vi "edge_trig_setup.vi"(7 "Tigger Level":dbl, 8 "error in (no error)":errorcluster, 9 "Coupling":u32(slide) scale=0.0..1.0, 10 "Channel":u32(slide)=1 scale=1.0..2.0, 11 "VISA In":refnum<visa-resource-name>) -> (0 "error out":errorcluster, 3 "VISA Out":refnum<visa-resource-name>)   [LabVIEW 2011]
panel:
  out "String Sent":string
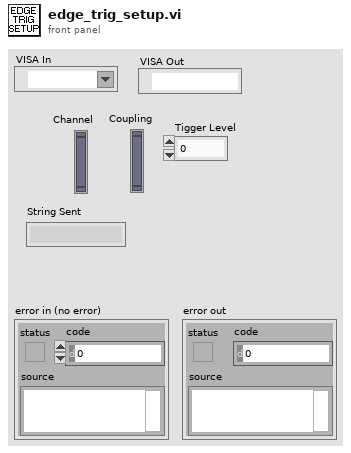
[diagram p1: front panel]
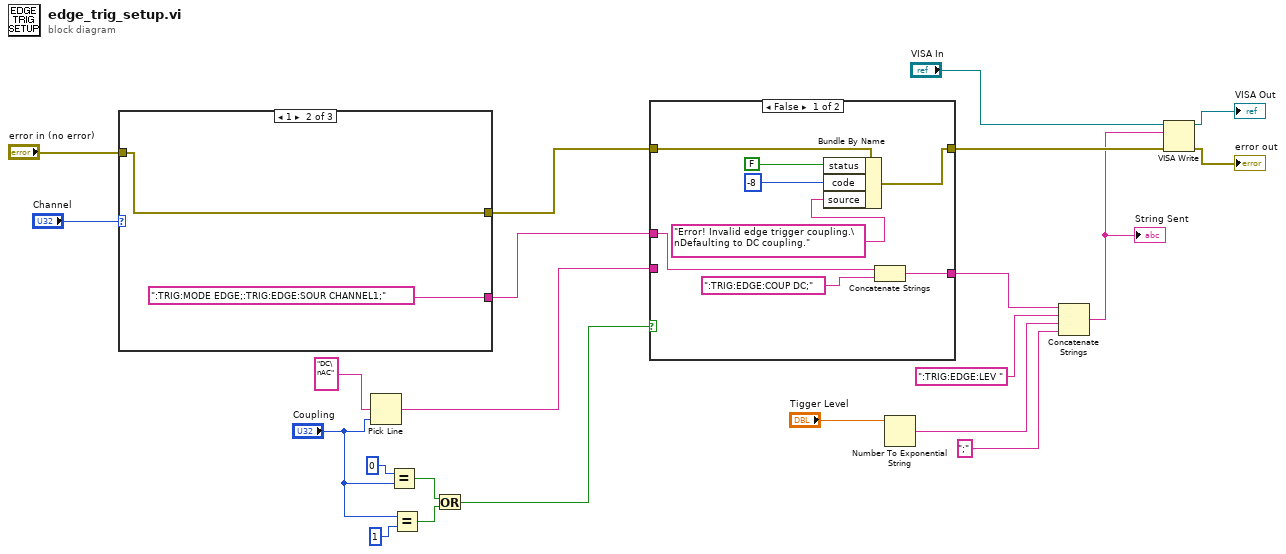
[diagram p0: block diagram]
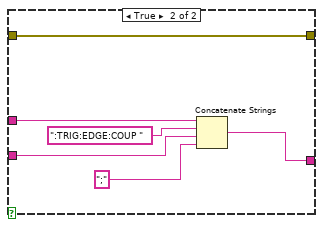
[diagram p2: hidden frame]
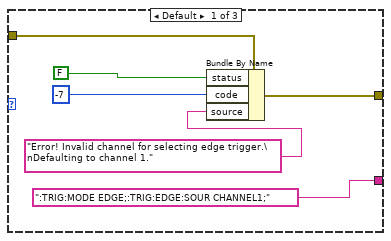
[diagram p3: hidden frame]
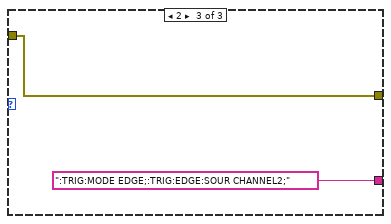
[diagram p4: hidden frame]
diagram:
  n1 = case shown="1" "Channel" {
    tunnel: "error in (no error)" -> [w28 w29 w31]
    tunnel: [w25 w29 w31] -> w18
    tunnel: [":TRIG:MODE EDGE;:TRIG:EDGE:SOUR CHANNEL1;" ":TRIG:MODE EDGE;:TRIG:EDGE:SOUR CHANNEL1;" ":TRIG:MODE EDGE;:TRIG:EDGE:SOUR CHANNEL2;"] -> w10
    frame Default {
      n2 = Bundle By Name(cluster=w28, "status"=FALSE, "code"=-7, "source"="Error! Invalid channel for selecting edge trigger.\nDefaulting to channel 1.") -> (w25:errorcluster)
    }
    frame 1 {
    }
    frame 2 {
    }
  }
  n3 = Pick Line(multi-line string="DC\nAC", line index="Coupling") -> (output string=w11:string)  [unwired: 1 in]
  n4 = Equal?(x=0, y="Coupling") -> (x = y?=w14:bool)
  n5 = Equal?(x="Coupling", y=1) -> (x = y?=w13:bool)
  n6 = Or(x=w14, y=w13) -> (x .or. y?=w12:bool)
  n7 = case shown="False" w12 {
    tunnel: w18 -> [w40 w46]
    tunnel: [w39 w46] -> w5
    tunnel: w11 -> [_ w43]
    tunnel: w10 -> [w34 w45]
    tunnel: [w33 w41] -> w9
    frame False {
      n8 = Bundle By Name(cluster=w40, "status"=FALSE, "code"=-8, "source"="Error! Invalid edge trigger coupling.\nDefaulting to DC coupling.") -> (w39:errorcluster)
      n9 = Concatenate Strings(w34, ":TRIG:EDGE:COUP DC;") -> (w33:string)
    }
    frame True {
      n10 = Concatenate Strings(w45, ":TRIG:EDGE:COUP ", w43, ";") -> (w41:string)
    }
  }
  n11 = Number To Exponential String(number="Tigger Level") -> (E-format string=w7:string)  [unwired: 3 in]
  n12 = Concatenate Strings(w9, ":TRIG:EDGE:LEV ", w7, ";") -> (w3:string)
  "String Sent" <- w3
  n13 = VISA Write(VISA resource name="VISA In", write buffer=w3, error in (no error)=w5) -> (VISA resource name out=→"VISA Out":refnum<visa-resource-name>, error out=→"error out":errorcluster)  [unwired: 1 out]
